vi "hmi_cheesy_drive_w_Help.vi"(9 "Quick Turn":bool, 10 "Wheel":dbl, 11 "Throttle":dbl) -> (3 "Drive Data":cluster{"Left":dbl, "Right":dbl})   [LabVIEW 2015]
doc: "Generates modified turn rates based on speed, steering wheel input, gear shift selection, and if \"Quick Turn\" is turned on. When \"Quick Turn\" is on faster turn rates are possible."
panel:
  in  "Speedturn_Sens_High":dbl=0.6
  in  "Speedturn_Sens_High max":dbl=0.6
  in  "Speedturn_Sens_Low max":dbl=0.6
  in  "gear shift state":enum16{"low", "high"}(ring)
  in  "Quickturn_Sens_High":dbl=1.0
  in  "Speedturn_Sens_Low":dbl=0.6
  in  "Quickturn_Sens_Low":dbl=1.0
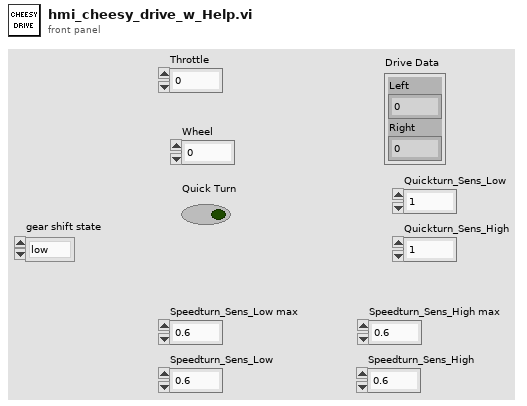
[diagram p1: front panel]
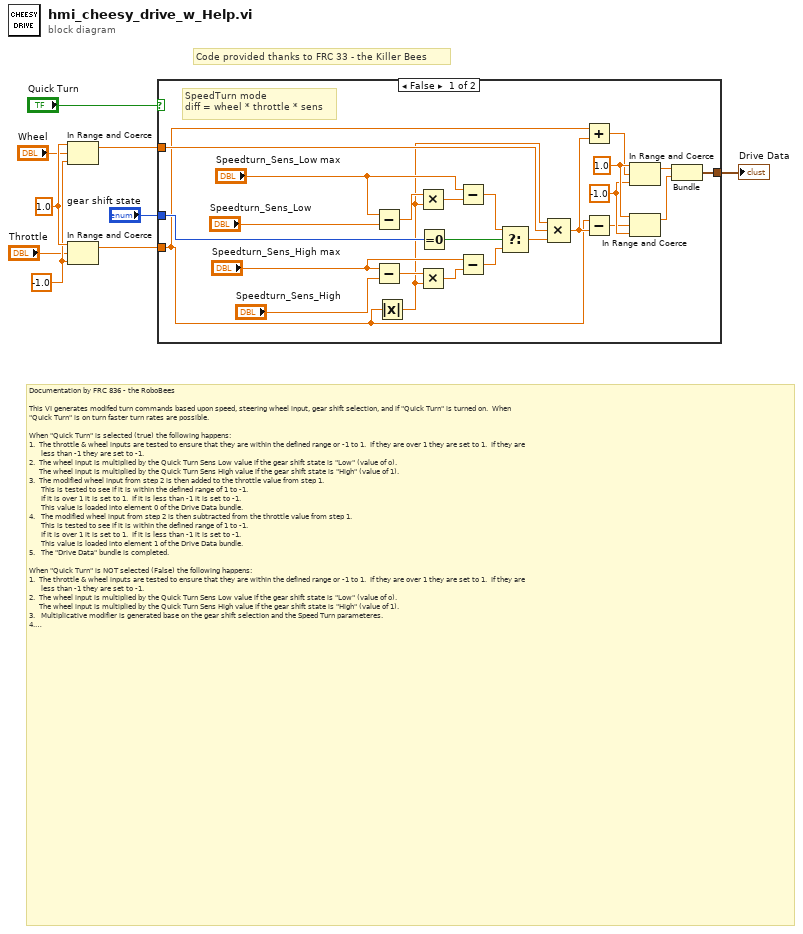
[diagram p0: block diagram]
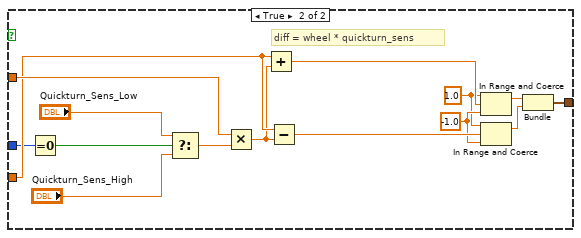
[diagram p2: hidden frame]
diagram:
  w5 = -1.0 ("lower limit")
  w6 = 1.0 ("upper limit")
  # "Documentation by FRC 836 - the RoboBees\n\nThis VI generates modifed turn commands based upon speed, steering wheel input, gear shift selection, and if \"Quick Turn\" is turned on.  When\n\"Quick Turn\" is on turn faster turn rates are possible.\n\nWhen \"Quick Turn\" is selected (true) the following happens:\n1.  The throttle & wheel inputs are tested to ensure that they are within the defined range or -1 to 1.  If they are over 1 they are set to 1.  If they are \n      less than -1 they are set to -1.\n2.  The wheel input is multiplied by the Quick Turn Sens Low value if the gear shift state is \"Low\" (value of o).\n     The wheel input is multiplied by the Quick Turn Sens High value if the gear shift state is \"High\" (value of 1).\n3.  The modified wheel input from step 2 is then added to the throttle value from step 1.\n      This is tested to see if it is within the defined range of 1 to -1.\n      If it is over 1 it is set to 1.  If it is less than -1 it is set to -1.\n      This value is loaded into element 0 of the Drive Data bundle.\n4.   The modified wheel input from step 2 is then subtracted from the throttle value from step 1.\n      This is tested to see if it is within the defined range of 1 to -1.\n      If it is over 1 it is set to 1.  If it is less than -1 it is set to -1.\n      This value is loaded into element 1 of the Drive Data bundle.\n5.   The \"Drive Data\" bundle is completed.\n\nWhen \"Quick Turn\" is NOT selected (False) the following happens:\n1.  The throttle & wheel inputs are tested to ensure that they are within the defined range or -1 to 1.  If they are over 1 they are set to 1.  If they are \n      less than -1 they are set to -1.\n2.  The wheel input is multiplied by the Quick Turn Sens Low value if the gear shift state is \"Low\" (value of o).\n     The wheel input is multiplied by the Quick Turn Sens High value if the gear shift state is \"High\" (value of 1).\n3.   Multiplicative modifier is generated base on the gear shift selection and the Speed Turn parameteres.\n4.   The modifer from step 3 is multipled with the wheel input and the absolute value of the throttle setting.\n5.   The output from step 4 is added to the throttle from step 1.\n      This is tested to see if it is within the defined range of 1 to -1.\n      If it is over 1 it is set to 1.  If it is less than -1 it is set to -1.\n      This value is loaded into element 0 of the Drive Data bundle.\n6.   The modified output from step 4 is then subtracted from the throttle value from step 1.\n      This is tested to see if it is within the defined range of 1 to -1.\n      If it is over 1 it is set to 1.  If it is less than -1 it is set to -1.\n      This value is loaded into element 1 of the Drive Data bundle.\n5.   The \"Drive Data\" bundle is completed."
  # "Code provided thanks to FRC 33 - the Killer Bees"
  n1 = In Range and Coerce(upper limit=w6, x="Wheel", lower limit=w5) -> (coerced(x)=w4:dbl)  [unwired: 1 out]
  n2 = In Range and Coerce(upper limit=w6, x="Throttle", lower limit=w5) -> (coerced(x)=w3:dbl)  [unwired: 1 out]
  n3 = case shown="False" "Quick Turn" {
    tunnel: w4 -> [w32 w44]
    tunnel: w3 -> [w20 w43]
    tunnel: [w10 w41] -> w9
    tunnel: "gear shift state" -> [w30 w40]
    frame False {
      w15 = -1.0 ("lower limit")
      w16 = 1.0 ("upper limit")
      # "SpeedTurn mode\ndiff = wheel * throttle * sens"
      n4 = Subtract(x="Speedturn_Sens_Low max", y="Speedturn_Sens_Low") -> (x-y=w27:dbl)
      n5 = Subtract(x="Speedturn_Sens_High max", y="Speedturn_Sens_High") -> (x-y=w22:dbl)
      n6 = Absolute Value(x=w20) -> (abs(x)=w17:dbl)
      n7 = Multiply(x=w27, y=w17) -> (x*y=w25:dbl)
      n8 = Multiply(x=w22, y=w17) -> (x*y=w24:dbl)
      n9 = Equal To 0?(x=w30) -> (x = 0?=w33:bool)
      n10 = Subtract(x="Speedturn_Sens_Low max", y=w25) -> (x-y=w18:dbl)
      n11 = Subtract(x="Speedturn_Sens_High max", y=w24) -> (x-y=w19:dbl)
      n12 = Select(t=w18, s=w33, f=w19) -> (s? t:f=w29:dbl)
      n13 = Compound Arithmetic op=MULTIPLY(w17, w32, w29) -> (w31:dbl)
      n14 = Add(x=w20, y=w31) -> (x+y=w14:dbl)
      n15 = Subtract(x=w20, y=w31) -> (x-y=w13:dbl)
      n16 = In Range and Coerce(upper limit=w16, x=w14, lower limit=w15) -> (coerced(x)=w11:dbl)  [unwired: 1 out]
      n17 = In Range and Coerce(upper limit=w16, x=w13, lower limit=w15) -> (coerced(x)=w12:dbl)  [unwired: 1 out]
      n18 = Bundle("upper limit"=w11, "upper limit"=w12) -> (w10:cluster{"upper limit":dbl, "upper limit":dbl})  [unwired: 1 in]
    }
    frame True {
      w35 = -1.0 ("lower limit")
      w34 = 1.0 ("upper limit")
      # "diff = wheel * quickturn_sens"
      n19 = Equal To 0?(x=w40) -> (x = 0?=w46:bool)
      n20 = Select(t="Quickturn_Sens_Low", s=w46, f="Quickturn_Sens_High") -> (s? t:f=w45:dbl)
      n21 = Multiply(x=w44, y=w45) -> (x*y=w42:dbl)
      n22 = Add(x=w43, y=w42) -> (x+y=w39:dbl)
      n23 = Subtract(x=w43, y=w42) -> (x-y=w37:dbl)
      n24 = In Range and Coerce(upper limit=w34, x=w39, lower limit=w35) -> (coerced(x)=w38:dbl)  [unwired: 1 out]
      n25 = In Range and Coerce(upper limit=w34, x=w37, lower limit=w35) -> (coerced(x)=w36:dbl)  [unwired: 1 out]
      n26 = Bundle("upper limit"=w38, "upper limit"=w36) -> (w41:cluster{"upper limit":dbl, "upper limit":dbl})  [unwired: 1 in]
    }
  }
  "Drive Data" <- w9
